vi "closeCAN_EPOS+DPS.vi"(8 "error in":errorcluster, 9 "DPS NodeID":u32[](array[numeric]), 10 "ObjHandle in":T1, 11 "axis in":cluster{"keyHandle":u32, "nodeId":u16}) -> (0 "error out":errorcluster)   [LabVIEW 2019]
uses:
  <vilib>/nican/nican.llb/xobjhandle.ctl
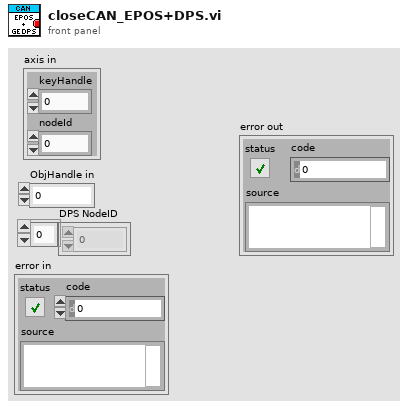
[diagram p1: front panel]
types:
  T1 = typedef "xobjhandle.ctl" = u32
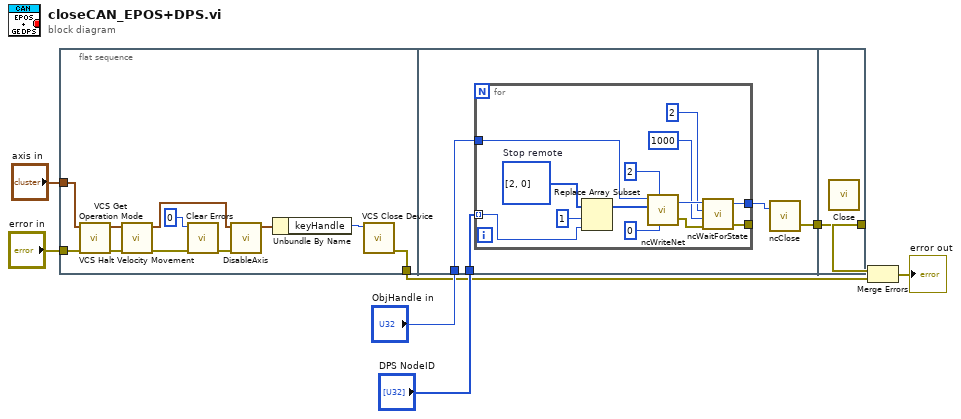
[diagram p0: block diagram]
diagram:
  n1 = flat-sequence {
    tunnel: "axis in" -> [w19]
    tunnel: "error in" -> [w18]
    tunnel: [w9] -> w3
    tunnel: "DPS NodeID" -> [w23]
    tunnel: "ObjHandle in" -> [w22]
    tunnel: [w20] -> w1
    tunnel: [w37] -> w4
    tunnel: w1 -> [w37]
    frame #0 {
      n2 = call <instrlib>:"VCS Get Operation Mode.vi"("error in (no error)"=w18, "axis in"=w19) -> ("error out"=w12:errorcluster, "axis out"=w13:cluster{"keyHandle":u32, "nodeId":u16})  [unwired: 7 in, 1 out]
      n3 = call <instrlib>:"VCS Halt Velocity Movement.vi"("error in (no error)"=w12, "axis in"=w13) -> ("error out"=w11:errorcluster, "axis out"=w10:cluster{"keyHandle":u32, "nodeId":u16})  [unwired: 8 in]
      n4 = call <vilib>:"Clear Errors.vi"("error in (no error)"=w11, "specific error code to clear (0: all)"=0) -> ("error out"=w17:errorcluster)  [unwired: 4 in, 1 out]
      n5 = call <instrlib>:"DisableAxis.vi"("error in (no error)"=w17, "axis in"=w10) -> ("axis out"=w15:cluster{"keyHandle":u32, "nodeId":u16})  [unwired: 4 in, 1 out]
      n6 = Unbundle By Name(w15) -> ("keyHandle"=w14:u32)
      n7 = call <instrlib>:"VCS Close Device.vi"("keyHandle in"=w14) -> ("error out"=w9:errorcluster)  [unwired: 10 in]
    }
    frame #1 {
      n8 = for {
        tunnel: w23 -> [w32] mode=indexing
        tunnel: w22 -> [w26]
        tunnel: [w24] -> _
        tunnel: [w25] -> w21
        w33 = u8[] [2, 0]  # Stop remote
        n9 = Replace Array Subset(array=w33, new element=w32, index=1) -> (w36:u8[])
        n10 = call <vilib>:"ncWriteNet.vi"("ArbitrationId"=u32 0, "DataLength"=u32 2, "Data"=w36, "ObjHandle in"=w26) -> ("Error out"=w35:errorcluster, "ObjHandle out"=w34:T1)  [unwired: 2 in]
        n11 = call <vilib>:"ncWaitForState.vi"("Error in"=w35, "Timeout"=u32 1000, "DesiredState"=u32 2, "ObjHandle in"=w34) -> ("Error out"=w24:errorcluster, "ObjHandle out"=w25:T1)  [unwired: 1 out]
      }
      n12 = call <vilib>:"ncClose.vi"("ObjHandle in"=w21) -> ("Error out"=w20:errorcluster)  [unwired: 2 in]
    }
    frame #2 {
      n13 = call <instrlib>:"Close.vi"() -> ()  [unwired: 11 in, 1 out]
    }
  }
  n14 = Merge Errors(w4, w3) -> (→"error out":errorcluster)
